vi "VIPM Post-Build Custom Action.vi"(10 "Variant":variant) -> (0 "error out":errorcluster)   [LabVIEW 2015]
uses:
  Program Files/National Instruments/LabVIEW 2023/user.lib/_OpenG.lib/appcontrol/appcontrol.llb/openg_application_control.lvlib
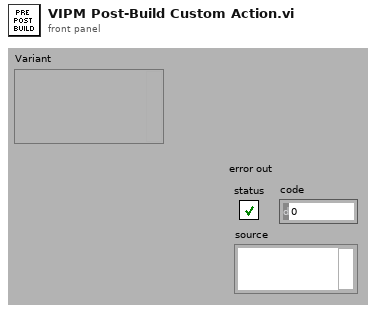
[diagram p1: front panel]
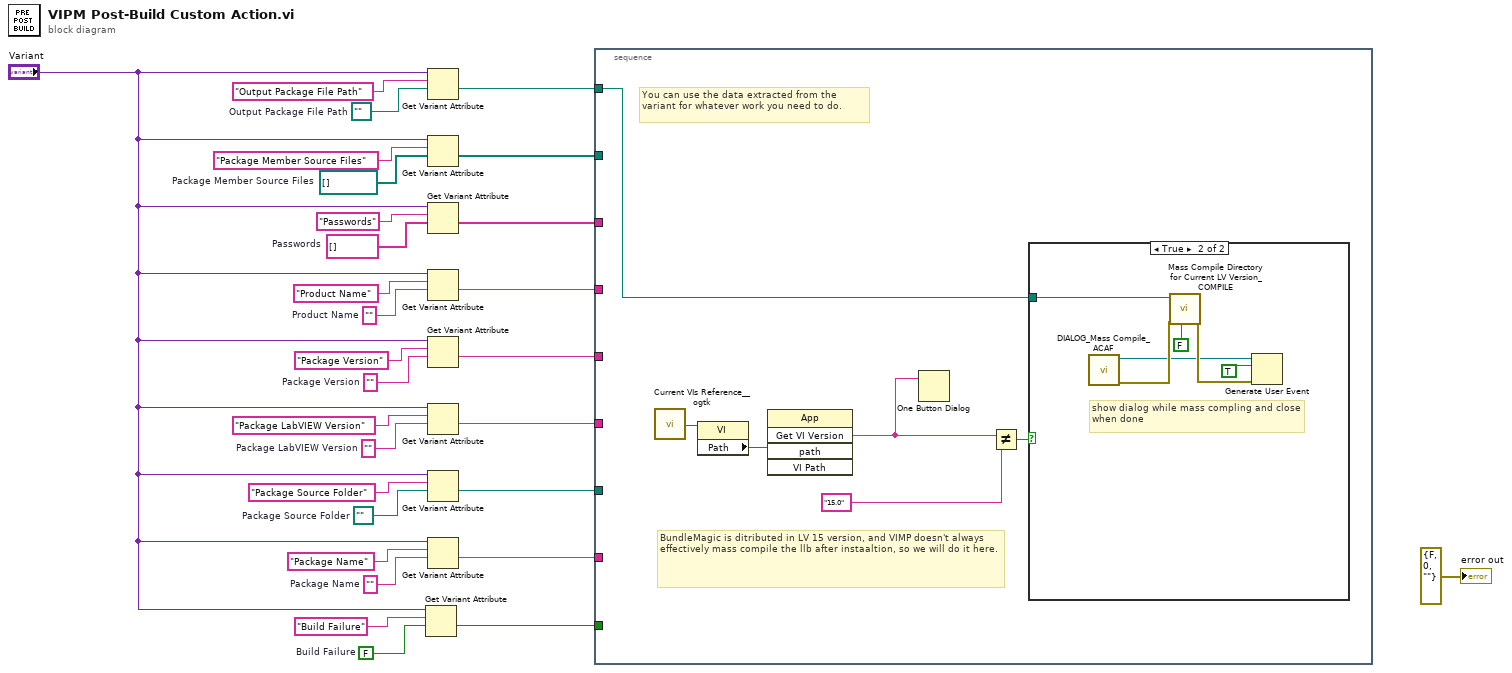
[diagram p0: block diagram]
diagram:
  w3 = FALSE  # Build Failure
  w13 = path ""  # Package Source Folder
  w14 = ""  # Package Name
  w17 = ""  # Package LabVIEW Version
  w19 = ""  # Package Version
  w21 = ""  # Product Name
  w24 = string[] []  # Passwords
  w26 = path[] []  # Package Member Source Files
  w28 = path ""  # Output Package File Path
  n1 = Get Variant Attribute(Variant="Variant", name="Build Failure", default value (empty Variant)=w3) -> (value=w1:bool)  [unwired: 1 in, 3 out]
  n2 = Get Variant Attribute(Variant="Variant", name="Output Package File Path", default value (empty Variant)=w28) -> (value=w12:path)  [unwired: 1 in, 3 out]
  n3 = Get Variant Attribute(Variant="Variant", name="Package Member Source Files", default value (empty Variant)=w26) -> (value=w11:path[])  [unwired: 1 in, 3 out]
  n4 = Get Variant Attribute(Variant="Variant", name="Passwords", default value (empty Variant)=w24) -> (value=w10:string[])  [unwired: 1 in, 3 out]
  n5 = Get Variant Attribute(Variant="Variant", name="Product Name", default value (empty Variant)=w21) -> (value=w9:string)  [unwired: 1 in, 3 out]
  n6 = Get Variant Attribute(Variant="Variant", name="Package Version", default value (empty Variant)=w19) -> (value=w8:string)  [unwired: 1 in, 3 out]
  n7 = Get Variant Attribute(Variant="Variant", name="Package LabVIEW Version", default value (empty Variant)=w17) -> (value=w7:string)  [unwired: 1 in, 3 out]
  n8 = Get Variant Attribute(Variant="Variant", name="Package Source Folder", default value (empty Variant)=w13) -> (value=w6:path)  [unwired: 1 in, 3 out]
  n9 = Get Variant Attribute(Variant="Variant", name="Package Name", default value (empty Variant)=w14) -> (value=w5:string)  [unwired: 1 in, 3 out]
  n10 = stacked-sequence {
    tunnel: w12 -> [w35]
    tunnel: w11 -> [_]
    tunnel: w10 -> [_]
    tunnel: w9 -> [_]
    tunnel: w8 -> [_]
    tunnel: w7 -> [_]
    tunnel: w6 -> [_]
    tunnel: w5 -> [_]
    tunnel: w1 -> [_]
    frame #0 {
      # "BundleMagic is ditributed in LV 15 version, and VIMP doesn't always effectively mass compile the llb after instaaltion, so we will do it here."
      # "You can use the data extracted from the variant for whatever work you need to do."
      n11 = call "Current VIs Reference__ogtk.vi"() -> ("Current VI's reference"=w34:refnum<vi>)  [unwired: 5 in]
      n12 = property class="VI"(reference=w34) -> ("Path"=w33:path)  [unwired: 1 in, 2 out]
      n13 = invoke class="App" method="Get VI Version"("path"=w33) -> ("GetVIVers"=w30:string)  [unwired: 4 in, 4 out]
      n14 = One Button Dialog(message=w30) -> ()  [unwired: 1 in, 1 out]
      n15 = Not Equal?(x=w30, y="15.0") -> (x != y?=w32:bool)
      n16 = case shown="True" w32 {
        tunnel: w35 -> [_ w41]
        frame False {
        }
        frame True {
          # "show dialog while mass compling and close when done"
          n17 = call "DIALOG_Mass Compile_ACAF.vi"() -> ("error out"=w39:errorcluster, "user event out"=w37:refnum<user-event>)  [unwired: 10 in]
          n18 = call "Mass Compile Directory for Current LV Version_COMPILE.vi"("List only Top-Level files in llbs? (FALSE)"=FALSE, "error in (no error)"=w39, "Folder of LabVIEW files to convert"=w41) -> ("error out"=w38:errorcluster)  [unwired: 8 in]
          n19 = Generate User Event(user event=w37, event data cluster=TRUE ("List only Top-Level files in llbs? (FALSE)"), error in=w38) -> ()  [unwired: 1 in, 2 out]
        }
      }
    }
  }
  "error out" <- errorcluster {"status"=FALSE, "code"=0, "source"=""} ("error out")
